vi "Agilent 66XX Series Take Measurement.vi"(0 "VISA resource name":refnum<visa-resource-name>, 1 "Preheat Current":dbl format="%.3f", 5 "Ouput(On:T)":bool=TRUE, 7 "Current Mode(Immediate:F)":bool, 9 "Voltage Mode(Immediate:F)":bool, 11 "error in (no error)":errorcluster, 12 "Voltage":dbl format="%.3f", 13 "Preheat Ramp Delay":u32=5000, 14 "Protection(None:0)":u16(ring) items=["None", "Overcurrent protection", "Overvoltage protection", "Overcurrent and overvoltage protection", "Clear overvoltage condition", "Clear overcurrent protection", "Set time delay"]) -> ()   [LabVIEW 2012]
doc: "The Application Example configures, triggers (after a user defined time delay) and stores the setting to a user defined address."
uses:
  Agilent 66XX Series.lvlib
panel:
  out "error out":errorcluster
  in  "Overvoltage prot value":dbl=5.0 format="%.3f"
  in  "Anneal Current":dbl format="%.3f"
  in  "Anneal Step Size":dbl format="%.3f"
  in  "Anneal Ramp Delay":u32=5000
  out "Anneal Current":dbl(graph)
  in  "Preheat Time":u32=5
  out "Preheat Current":dbl(graph)
  in  "START":bool
  in  "Preheat Step Size":dbl format="%.3f"
  in  "Reset (F:no)":bool
  in  "ID query (T:yes)":bool=TRUE
  # "Power Supply Configurations"
  # "Preheat Settings"
  # "Amps"
  # "min"
  # "Amps/Step"
  # "ms"
  # "Anneal Settings"
  # "Yes"
  # "No"
  # "Yes"
  # "No"
  # "Trigger"
  # "Immediate"
  # "Trigger"
  # "Immediate"
  # "On"
  # "Off"
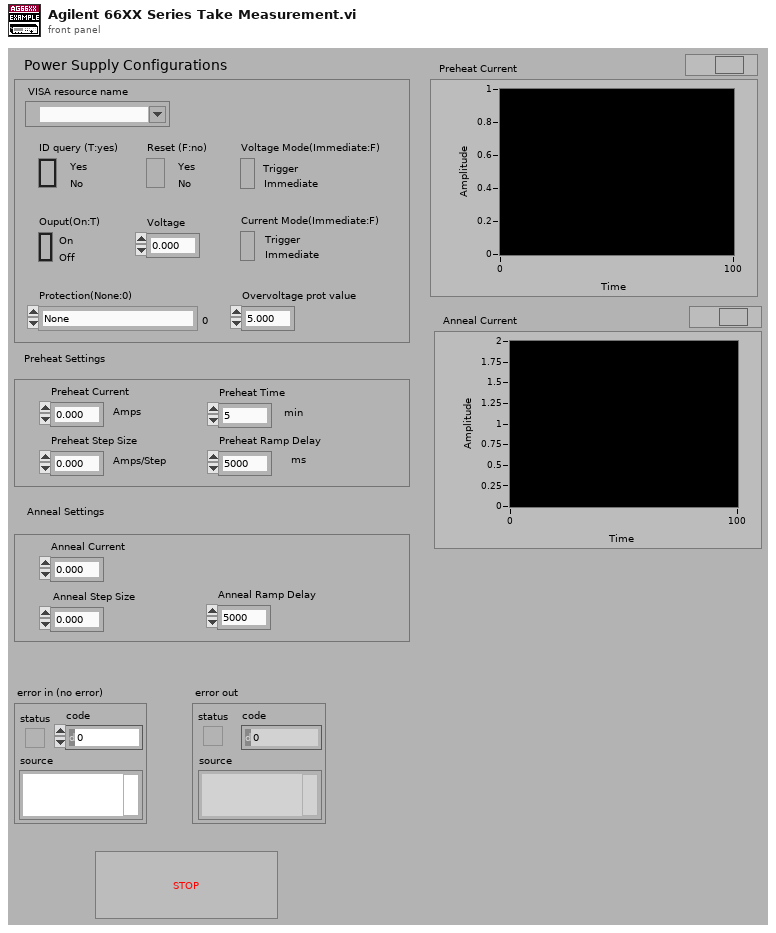
[diagram p1: front panel]
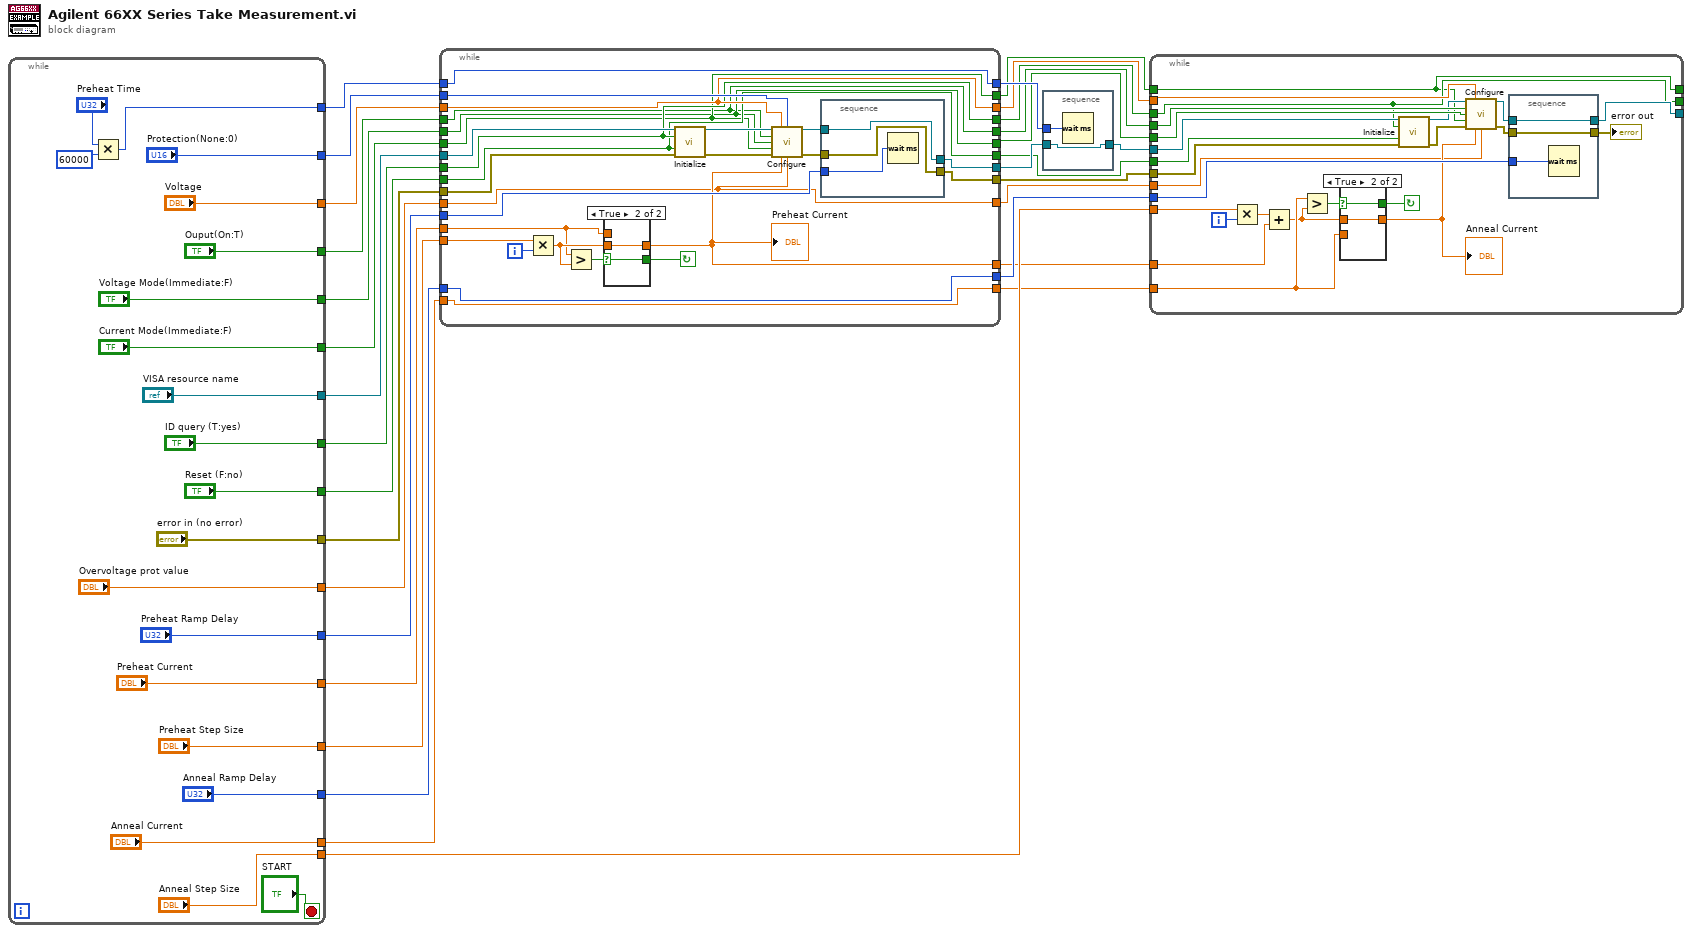
[diagram p0: block diagram]
diagram:
  n1 = while {
    tunnel: ["Current Mode(Immediate:F)"] -> w31
    tunnel: ["Voltage Mode(Immediate:F)"] -> w30
    tunnel: ["Ouput(On:T)"] -> w29
    tunnel: ["Voltage"] -> w28
    tunnel: ["Protection(None:0)"] -> w27
    tunnel: ["Preheat Current"] -> w26
    tunnel: ["Preheat Ramp Delay"] -> w25
    tunnel: ["VISA resource name"] -> w24
    tunnel: ["ID query (T:yes)"] -> w23
    tunnel: ["Reset (F:no)"] -> w22
    tunnel: ["error in (no error)"] -> w21
    tunnel: ["Preheat Step Size"] -> w20
    tunnel: [w32] -> w18
    tunnel: ["Anneal Ramp Delay"] -> w16
    tunnel: ["Anneal Step Size"] -> w10
    tunnel: ["Anneal Current"] -> w8
    tunnel: ["Overvoltage prot value"] -> w2
    stop <- "START" stop-if-true
    n2 = Multiply(x="Preheat Time", y=60000) -> (x*y=w32:u32)
  }
  n3 = while {
    tunnel: w31 -> [w56]
    tunnel: w30 -> [w55]
    tunnel: w29 -> [w54]
    tunnel: w28 -> [w63]
    tunnel: w27 -> [w78]
    tunnel: w26 -> [w68]
    tunnel: w25 -> [w76]
    tunnel: w24 -> [w62]
    tunnel: w23 -> [w61]
    tunnel: w22 -> [w60]
    tunnel: w21 -> [w73]
    tunnel: w20 -> [w71]
    tunnel: [w66] -> w19
    tunnel: [w65] -> w17
    tunnel: w18 -> [w65]
    tunnel: w16 -> [w64]
    tunnel: [w64] -> w15
    tunnel: [w63] -> w14
    tunnel: [w61] -> w13
    tunnel: [w60] -> w12
    tunnel: [w59] -> w11
    tunnel: [w58] -> w9
    tunnel: w8 -> [w57]
    tunnel: [w57] -> w7
    tunnel: [w56] -> w5
    tunnel: [w55] -> w4
    tunnel: [w54] -> w3
    tunnel: w2 -> [w52]
    tunnel: [w52] -> w1
    i -> [w72]
    stop <- w67 continue-if-true
    n4 = Multiply(x=w71, y=w72) -> (x*y=w69:dbl)
    n5 = Greater?(x=w68, y=w69) -> (0:w70:bool)
    n6 = case shown="True" w70 {
      selector: w70 -> [w79 w81]
      tunnel: w69 -> [_ w82]
      tunnel: [w80 w82] -> w58
      tunnel: w68 -> [w80 _]
      tunnel: [w79 w81] -> w67
      frame False {
      }
      frame True {
      }
    }
    "Preheat Current" <- w58
    n7 = call "Initialize.vi"("VISA resource name"=w62, "ID query (T:yes)"=w61, "Reset (F:no)"=w60, "error in (no error)"=w73) -> ("VISA resource name out"=w75:refnum<visa-resource-name>, "error out"=w74:errorcluster)  [unwired: 10 in]
    n8 = call "Configure.vi"("VISA resource name"=w75, "Voltage(0 Volts)"=w63, "Protection(None:0)"=w78, "Ouput(On:T)"=w54, "Voltage Mode(F:Immediate)"=w55, "Current Mode(F:Immediate)"=w56, "error in (no error)"=w74, "Current(0 Amps)"=w58, "Overvoltage prot value(50 Volts)"=w52) -> ("VISA resource name out"=w77:refnum<visa-resource-name>, "error out"=w53:errorcluster)  [unwired: 5 in]
    n9 = stacked-sequence {
      tunnel: w77 -> [w85]
      tunnel: w53 -> [w84]
      tunnel: [w85] -> w66
      tunnel: [w84] -> w59
      tunnel: w76 -> [w83]
      frame #0 {
        n10 = Wait (ms)(milliseconds to wait=w83) -> ()  [unwired: 1 out]
      }
    }
  }
  n11 = stacked-sequence {
    tunnel: w19 -> [w87]
    tunnel: [w87] -> w6
    tunnel: w17 -> [w86]
    frame #0 {
      n12 = Wait (ms)(milliseconds to wait=w86) -> ()  [unwired: 1 out]
    }
  }
  n13 = while {
    tunnel: [w90] -> _
    tunnel: w4 -> [w112]
    tunnel: w3 -> [w111]
    tunnel: w14 -> [w110]
    tunnel: w7 -> [w99]
    tunnel: w15 -> [w107]
    tunnel: w6 -> [w104]
    tunnel: [w95] -> _
    tunnel: w12 -> [w103]
    tunnel: w10 -> [w101]
    tunnel: [w96] -> _
    tunnel: w13 -> [w95]
    tunnel: w11 -> [w94]
    tunnel: w9 -> [w92]
    tunnel: w5 -> [w90]
    tunnel: w1 -> [w88]
    i -> [w102]
    stop <- w98 continue-if-true
    n14 = Multiply(x=w101, y=w102) -> (x*y=w93:dbl)
    n15 = Add(x=w93, y=w92) -> (x+y=w91:dbl)
    n16 = Greater?(x=w99, y=w91) -> (0:w100:bool)
    n17 = case shown="True" w100 {
      selector: w100 -> [w113 w115]
      tunnel: w91 -> [_ w116]
      tunnel: [w114 w116] -> w97
      tunnel: w99 -> [w114 _]
      tunnel: [w113 w115] -> w98
      frame False {
      }
      frame True {
      }
    }
    "Anneal Current" <- w97
    n18 = call "Initialize.vi"("VISA resource name"=w104, "ID query (T:yes)"=w95, "Reset (F:no)"=w103, "error in (no error)"=w94) -> ("VISA resource name out"=w106:refnum<visa-resource-name>, "error out"=w105:errorcluster)  [unwired: 10 in]
    n19 = call "Configure.vi"("VISA resource name"=w106, "Voltage(0 Volts)"=w110, "Ouput(On:T)"=w111, "Voltage Mode(F:Immediate)"=w112, "Current Mode(F:Immediate)"=w90, "error in (no error)"=w105, "Current(0 Amps)"=w97, "Overvoltage prot value(50 Volts)"=w88) -> ("VISA resource name out"=w109:refnum<visa-resource-name>, "error out"=w108:errorcluster)  [unwired: 6 in]
    n20 = stacked-sequence {
      tunnel: w109 -> [w119]
      tunnel: w108 -> [w118]
      tunnel: [w119] -> w96
      tunnel: [w118] -> w89
      tunnel: w107 -> [w117]
      frame #0 {
        n21 = Wait (ms)(milliseconds to wait=w117) -> ()  [unwired: 1 out]
      }
    }
    "error out" <- w89
  }
